vi "Singlent(SubVI).vi"(4 "Trigger Level (0.0 V)":dbl, 5 "Source (1: Channel 1)":u16(ring)=1 items=["Channel 1"=1, "Channel 2"=2, "Channel 3"=3, "Channel 4"=4], 6 "Timebase (0.0005 s)":dbl=0.2, 7 "Vertical Coupling (0: A1M)":u16(ring)=2 items=["A1M", "A50", "D1M", "D50", "Ground"], 8 "Vertical Range (1 V)":dbl=2.0, 9 "Probe Attenuation (1X)":dbl=1.0, 10 "length":i32=1044000, 11 "VISA Refnum in":refnum<visa-resource-name>="USB0::0xF4EC::0xEE38::SDSMMEBX3R2562::INSTR") -> (3 "Waveform Graph":waveform(dbl))   [LabVIEW 2018]
uses:
  <instrlib>/Siglent SDS 1000 2000 Series/Public/Configure/Configure Trigger (Edge).vi
  <instrlib>/Siglent SDS 1000 2000 Series/Public/Data/Read Waveform (Single).vi
  <instrlib>/Siglent SDS 1000 2000 Series/Siglent SDS 1000 2000 Series.lvlib
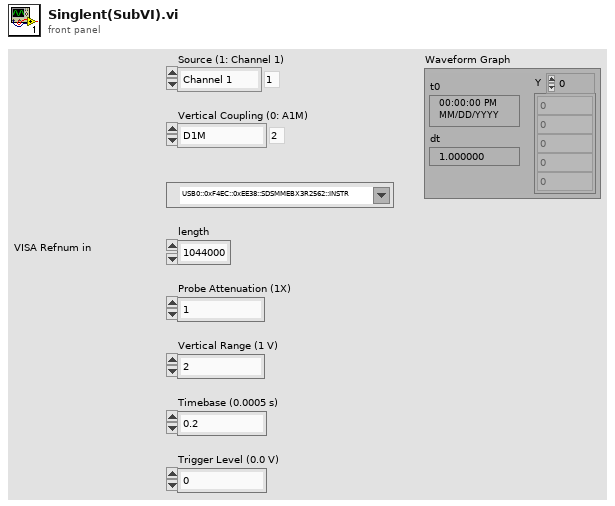
[diagram p1: front panel]
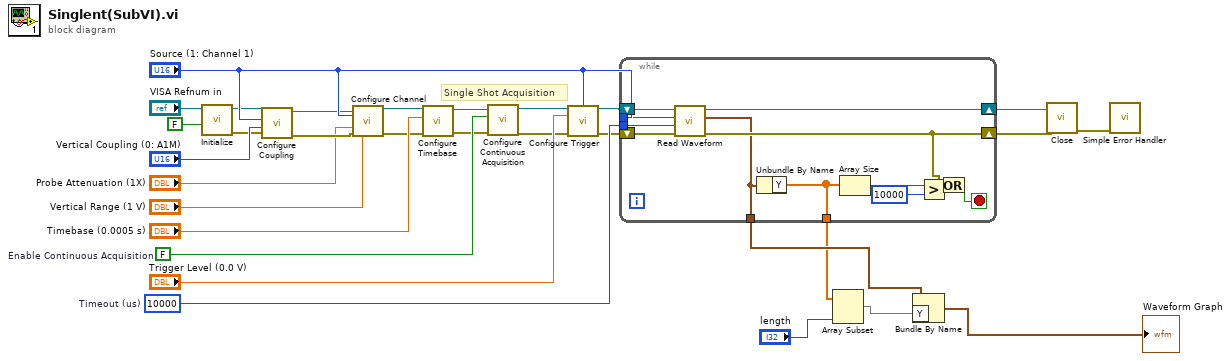
[diagram p0: block diagram]
diagram:
  w18 = u32 10000  # Timeout (us)
  w15 = FALSE  # Enable Continuous Acquisition
  # "Single Shot Acquisition"
  n1 = call <instrlib>:"Initialize.vi"("Reset (True)"=FALSE ("Reset? (T: Yes)"), "VISA resource name"="VISA Refnum in") -> ("error out"=w23:errorcluster, "VISA resource name out"=w20:refnum<visa-resource-name>)  [unwired: 8 in]
  n2 = call <instrlib>:"Configure Coupling.vi"("error in (no error)"=w23, "Vertical Coupling (0: A1M)"="Vertical Coupling (0: A1M)", "Channel (1: Channel 1)"="Source (1: Channel 1)", "VISA resource name"=w20) -> ("error out"=w22:errorcluster, "VISA resource name out"=w21:refnum<visa-resource-name>)  [unwired: 6 in]
  n3 = call <instrlib>:"Configure Channel.vi"("VISA resource name"=w21, "Channel (1: Channel 1)"="Source (1: Channel 1)", "Probe Attenuation (1X)"="Probe Attenuation (1X)", "error in (no error)"=w22, "Vertical Range (1.0 V)"="Vertical Range (1 V)") -> ("VISA resource name out"=w3:refnum<visa-resource-name>, "error out"=w2:errorcluster)  [unwired: 9 in]
  n4 = call <instrlib>:"Configure Timebase.vi"("error in (no error)"=w2, "Timebase (0.0005 s)"="Timebase (0.0005 s)", "VISA resource name"=w3) -> ("error out"=w13:errorcluster, "VISA resource name out"=w10:refnum<visa-resource-name>)  [unwired: 7 in]
  n5 = call <instrlib>:"Configure Continuous Acquisition.vi"("error in (no error)"=w13, "Enable Continuous Acquisition(T: On)"=w15, "VISA resource name"=w10) -> ("error out"=w12:errorcluster, "VISA resource name out"=w11:refnum<visa-resource-name>)  [unwired: 7 in]
  n6 = call-poly <instrlib>:"Configure Trigger.vi"("VISA resource name"=w11, "Trigger Source (1: Channel 1)"="Source (1: Channel 1)", "Trigger Level (0.0 V)"="Trigger Level (0.0 V)", "error in (no error)"=w12) -> ("VISA resource name out"=w8:refnum<visa-resource-name>, "error out"=w9:errorcluster)  [unwired: 10 in]
  n7 = while {
    tunnel: w18 -> [w39]
    tunnel: "Source (1: Channel 1)" -> [w38]
    shift-right: [w42] -> w6
    shift-left: w8 -> [w41]
    shift-right: [w32] -> w7
    shift-left: w9 -> [w40]
    tunnel: [w37] -> w27
    tunnel: [w31] -> w29
    stop <- w33 stop-if-true
    n8 = call-poly <instrlib>:"Read Waveform.vi"("error in (no error)"=w40, "Timeout (10000 ms)"=w39, "Source (1: Channel 1)"=w38, "VISA resource name"=w41) -> ("error out"=w32:errorcluster, "Waveform Graph"=w31:waveform(dbl), "VISA resource name out"=w42:refnum<visa-resource-name>)  [unwired: 5 in]
    n9 = Unbundle By Name(w31) -> ("Y"=w37:dbl[])
    n10 = Array Size(array=w37) -> (size(s)=w35:i32)
    n11 = Greater?(x=w35, y=10000) -> (0:w36:bool)
    n12 = Or(x=w32, y=w36) -> (x .or. y?=w33:bool)
  }
  n13 = Array Subset(array=w27, length="length") -> (w28:dbl[])  [unwired: 1 in]
  n14 = Bundle By Name(cluster=w29, "Y"=w28) -> (→"Waveform Graph":waveform(dbl))
  n15 = call <instrlib>:"Close.vi"("error in (no error)"=w7, "VISA resource name"=w6) -> ("error out"=w1:errorcluster)  [unwired: 9 in]
  n16 = call <vilib>:"Simple Error Handler.vi"("error in (no error)"=w1) -> ()  [unwired: 4 in, 5 out]
